vi "Dispose(冲突时的文件备份2013-05-03 10-15-52).vi"(8 "错误输入（无错误）":errorcluster, 10 "事件注册引用句柄":refnum<k27>, 11 "Filesytem Watcher Ref":refnum<k24>) -> (0 "错误输出":errorcluster)   [LabVIEW 2012, in "FileSystem Watcher.lvlib"]
uses:
  FileSystem Watcher.lvlib
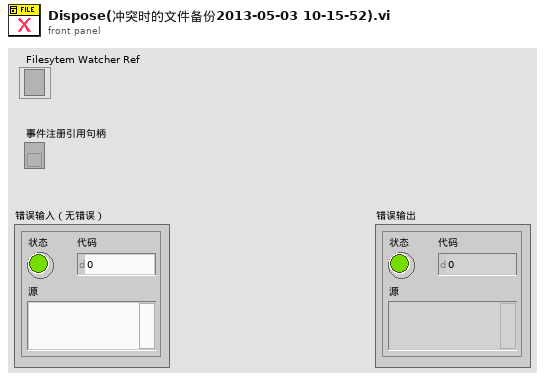
[diagram p1: front panel]
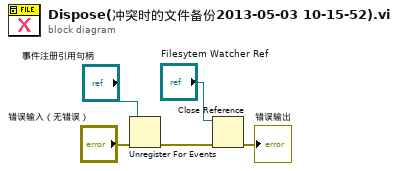
[diagram p0: block diagram]
diagram:
  n1 = Unregister For Events(event registration refnum="事件注册引用句柄", error in="错误输入（无错误）") -> (error out=w1:errorcluster)
  n2 = Close Reference(reference="Filesytem Watcher Ref", error in (no error)=w1) -> (error out=→"错误输出":errorcluster)
